vi "Send GOODBYE.vi"(8 "timeout ms (100)":i32=100, 9 "Goodbye Request":T1={"Error URI"="wamp.error.protocol_violation", "Message"=""}, 10 "error in (no error)":errorcluster, 11 "WAMP Client in":refnum<class "WAMP Client.lvclass">) -> (2 "error out":errorcluster, 3 "WAMP Client out":refnum<class "WAMP Client.lvclass">)   [LabVIEW 2020, in "WAMP Client.lvclass"]
uses:
  <userlib>/lvwamp/WAMP Client/WAMP Client.lvclass
  <userlib>/lvwamp/WAMP Client/TypeDef/GOODBYE Request Data.ctl
  <userlib>/lvwamp/WAMP Client/WAMP Client.lvclass/WAMP Client.ctl
  <userlib>/lvwamp/Comm Handlers/ICommHandler/ICommHandler.lvclass
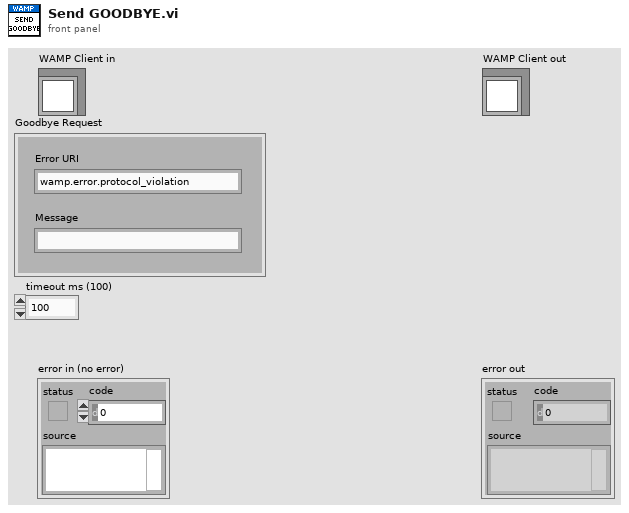
[diagram p1: front panel]
types:
  T1 = typedef "WAMP Client.lvclass/GOODBYE Request Data.ctl" = cluster{"Error URI":string, "Message":string}
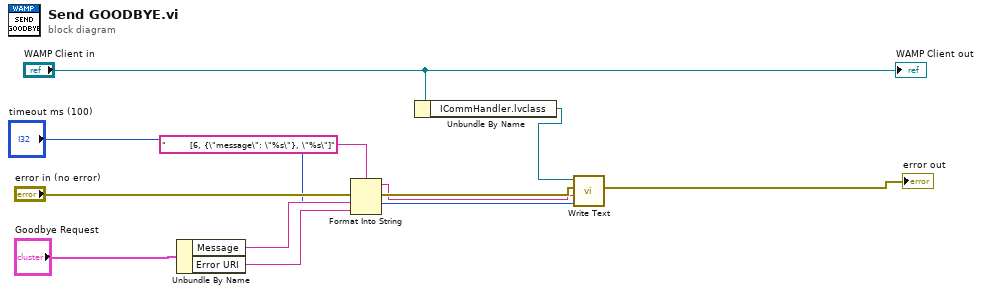
[diagram p0: block diagram]
diagram:
  n1 = Unbundle By Name("Goodbye Request") -> ("Message"=w10:string, "Error URI"=w9:string)
  n2 = Format Into String(format string="        [6, {\"message\": \"%s\"}, \"%s\"]", error in="error in (no error)", w10, w9) -> (resulting string=w3:string, error out=w4:errorcluster)  [unwired: 1 in]
  n3 = Unbundle By Name("WAMP Client in") -> ("ICommHandler.lvclass"=w5:refnum<class "ICommHandler.lvclass">)
  n4 = call-dynamic "Write Text.vi"("timeout ms (5000)"="timeout ms (100)", "String"=w3, "error in (no error)"=w4, "ICommHandler in"=w5) -> ("error out"=→"error out":errorcluster)  [unwired: 6 in, 1 out]
  "WAMP Client out" <- "WAMP Client in"
